vi "ws_set_target.vi"(0 "name":string, 1 "pool0":string, 2 "pool1":string, 3 "pool2":string, 5 "in_use":bool, 7 "user":string, 9 "procs":u16, 11 "os":string, 12 "tag0":string, 13 "tag1":string, 14 "tag2":string) -> (4 "success":bool, 10 "Error?":bool, 15 "Error_info":string)   [LabVIEW 2011]
uses:
  CommonTargetData.ctl
panel:
  in  "CommonTargetData":T1
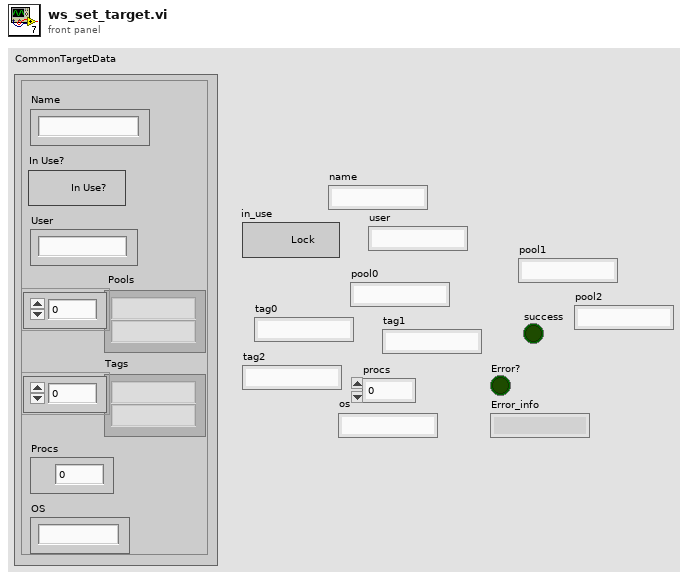
[diagram p1: front panel]
types:
  T1 = typedef "CommonTargetData.ctl" = cluster{"Name":string, "In Use?":bool, "User":string, " Pools":string[], "Tags":string[], "Procs":u16, "OS":string}
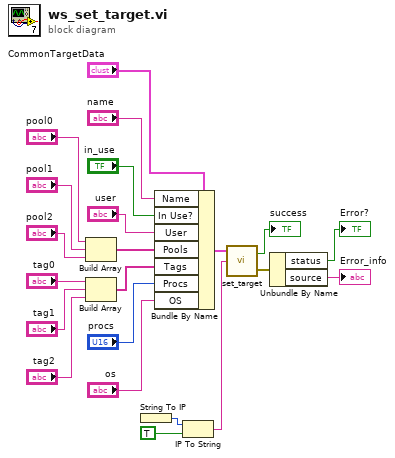
[diagram p0: block diagram]
diagram:
  n1 = Build Array("pool0", "pool1", "pool2") -> (w1:string[])
  n2 = Build Array("tag0", "tag1", "tag2") -> (w5:string[])
  n3 = String To IP() -> (0:w22:u32)  [unwired: 1 in]
  n4 = Bundle By Name(cluster="CommonTargetData", "Name"="name", "In Use?"="in_use", "User"="user", "Pools"=w1, "Tags"=w5, "Procs"="procs", "OS"="os") -> (w17:T1)
  n5 = IP To String(1:TRUE ("dot notation? (F)"), 2:w22) -> (0:w15:string)
  n6 = call "set_target.vi"("Remote Server Address"=w15, "CommonTargetData"=w17) -> ("error out"=w14:errorcluster, "success"=→"success":bool)  [unwired: 1 in]
  n7 = Unbundle By Name(w14) -> ("status"=→"Error?":bool, "source"=→"Error_info":string)
